vi "RFID GlobalVariable.vi"() -> ()   [LabVIEW 2018]
uses:
  Return_t.ctl
panel:
  out "_head":u16
  out "opcode Rd":u8 format="%x"
  out "crc Rd":u16=7439 format="%x"
  out "messageLength Rd":u8
  out "Wr Array":string[](array[string])
  out "msg read":u8[](array[numeric]) format="%x"
  in  "Tag Protocol":u16(ring)=5 items=["TMR_TAG_PROTOCOL_NONE"=0, "TMR_TAG_PROTOCOL_ISO180006B"=3, "TMR_TAG_PROTOCOL_GEN2"=5, "TMR_TAG_PROTOCOL_ISO180006B_UCODE"=6, "TMR_TAG_PROTOCOL_IPX64"=7, "TMR_TAG_PROTOCOL_IPX256"=8, "TMR_TAG_PROTOCOL_ATA"=29]
  in  "Region":u16(ring)=8 items=["REGION_INDIA"=4, "REGION_JAPAN"=5, "REGION_CHINA"=6, "REGION_EUROPE"=8, "REGION_KOREA"=9, "REGION_AUSTRALIA"=11, "REGION_NEWZEALAND"=13, "REGION_OPEN"=255]
  in  "Cmd_Time_Out":u16(ring)=2000 items=["COMMAND_TIME_OUT"=2000]
  in  "Opcode Constant":u16(ring) items=["TMR_SR_OPCODE_VERSION"=3, "TMR_SR_OPCODE_SET_BAUD_RATE"=6, "TMR_SR_OPCODE_READ_TAG_ID_SINGLE"=33, "TMR_SR_OPCODE_READ_TAG_ID_MULTIPLE"=34, "TMR_SR_OPCODE_WRITE_TAG_ID"=35, "TMR_SR_OPCODE_WRITE_TAG_DATA"=36, "TMR_SR_OPCODE_KILL_TAG"=38, "TMR_SR_OPCODE_READ_TAG_DATA"=40, "TMR_SR_OPCODE_CLEAR_TAG_ID_BUFFER"=42, "TMR_SR_OPCODE_MULTI_PROTOCOL_TAG_OP"=47, "TMR_SR_OPCODE_GET_READ_TX_POWER"=98, "TMR_SR_OPCODE_GET_WRITE_TX_POWER"=100, "TMR_SR_OPCODE_GET_POWER_MODE"=104, "TMR_SR_OPCODE_GET_READER_OPTIONAL_PARAMS"=106, "TMR_SR_OPCODE_GET_PROTOCOL_PARAM"=107, "TMR_SR_OPCODE_SET_ANTENNA_PORT"=145, "TMR_SR_OPCODE_SET_TAG_PROTOCOL"=147, "TMR_SR_OPCODE_SET_READ_TX_POWER"=146, "TMR_SR_OPCODE_SET_WRITE_TX_POWER"=148, "TMR_SR_OPCODE_SET_REGION"=151, "TMR_SR_OPCODE_SET_READER_OPTIONAL_PARAMS"=154, "TMR_SR_OPCODE_SET_PROTOCOL_PARAM"=155]
  in  "Return":T1
  out "opcode":u8 format="%x"
  out "crc":u16=7439 format="%x"
  out "messageLength":u8
  out "msg":u8[](array[numeric]) format="%x"
  # "Need only \nto debugging.\n<Arry of strings>"
  # "#define TMR_SR_OPCODE_VERSION 0x03\n#define TMR_SR_OPCODE_SET_BAUD_RATE 0x06\n#define TMR_SR_OPCODE_READ_TAG_ID_SINGLE 0x21\n#define TMR_SR_OPCODE_READ_TAG_ID_MULTIPLE 0x22\n#define TMR_SR_OPCODE_WRITE_TAG_ID 0x23\n#define TMR_SR_OPCODE_WRITE_TAG_DATA 0x24\n#define TMR_SR_OPCODE_KILL_TAG 0x26\n#define TMR_SR_OPCODE_READ_TAG_DATA 0x28\n#define TMR_SR_OPCODE_CLEAR_TAG_ID_BUFFER 0x2A\n#define TMR_SR_OPCODE_MULTI_PROTOCOL_TAG_OP 0x2F\n#define TMR_SR_OPCODE_GET_READ_TX_POWER 0x62\n#define TMR_SR_OPCODE_GET_WRITE_TX_POWER 0x64\n#define TMR_SR_OPCODE_GET_POWER_MODE 0x68\n#define TMR_SR_OPCODE_GET_READER_OPTIONAL_PARAMS 0x6A\n#define TMR_SR_OPCODE_GET_PROTOCOL_PARAM 0x6B\n#define TMR_SR_OPCODE_SET_ANTENNA_PORT 0x91\n#define TMR_SR_OPCODE_SET_TAG_PROTOCOL 0x93\n#define TMR_SR_OPCODE_SET_READ_TX_POWER 0x92\n#define TMR_SR_OPCODE_SET_WRITE_TX_POWER 0x94\n#define TMR_SR_OPCODE_SET_REGION 0x97\n#define TMR_SR_OPCODE_SET_READER_OPTIONAL_PARAMS 0x9A\n#define TMR_SR_OPCODE_SET_PROTOCOL_PARAM 0x9B"
  # "//Define all the ways functions can return\n#define ALL_GOOD 0\n#define ERROR_COMMAND_RESPONSE_TIMEOUT 1\n#define ERROR_CORRUPT_RESPONSE 2\n#define ERROR_WRONG_OPCODE_RESPONSE 3\n#define ERROR_UNKNOWN_OPCODE 4\n#define RESPONSE_IS_TEMPERATURE 5\n#define RESPONSE_IS_KEEPALIVE 6\n#define RESPONSE_IS_TEMPTHROTTLE 7\n#define RESPONSE_IS_TAGFOUND 8\n#define RESPONSE_IS_NOTAGFOUND 9\n#define RESPONSE_IS_UNKNOWN 10\n#define RESPONSE_SUCCESS 11\n#define RESPONSE_FAIL 12"
  # "#define REGION_INDIA 0x04\n#define REGION_JAPAN 0x05\n#define REGION_CHINA 0x06\n#define REGION_EUROPE 0x08\n#define REGION_KOREA 0x09\n#define REGION_AUSTRALIA 0x0B\n#define REGION_NEWZEALAND 0x0C\n#define REGION_NORTHAMERICA 0x0D\n#define REGION_OPEN 0xFF"
  # "//and possible future support\n//TMR_TAG_PROTOCOL_NONE              = 0x00\n//TMR_TAG_PROTOCOL_ISO180006B        = 0x03\n//TMR_TAG_PROTOCOL_GEN2              = 0x05\n//TMR_TAG_PROTOCOL_ISO180006B_UCODE  = 0x06\n//TMR_TAG_PROTOCOL_IPX64             = 0x07\n//TMR_TAG_PROTOCOL_IPX256            = 0x08\n//TMR_TAG_PROTOCOL_ATA               = 0x1D"
  # "#define COMMAND_TIME_OUT 2000"
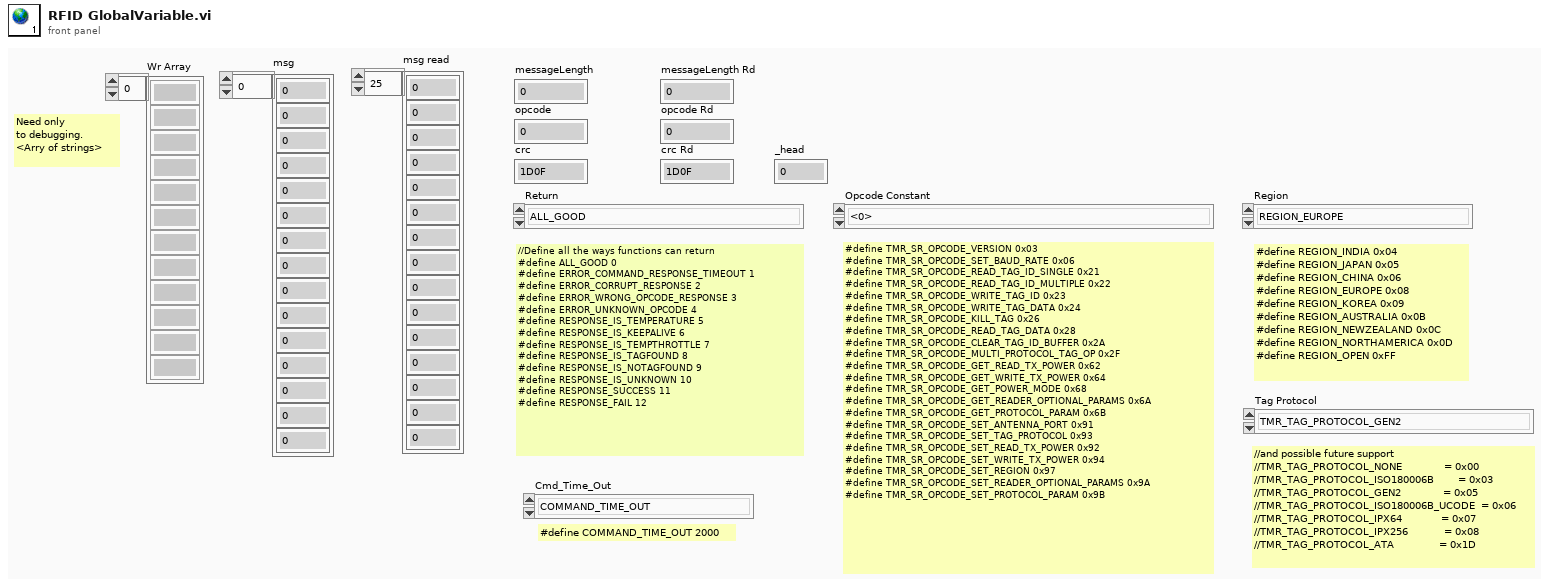
[diagram p1: front panel]
types:
  T1 = typedef "Return_t.ctl" = enum16{"ALL_GOOD", "ERROR_COMMAND_RESPONSE_TIMEOUT", "ERROR_CORRUPT_RESPONSE", "ERROR_WRONG_OPCODE_RESPONSE", "ERROR_UNKNOWN_OPCODE", "RESPONSE_IS_TEMPERATURE", "RESPONSE_IS_KEEPALIVE", "RESPONSE_IS_TEMPTHROTTLE", "RESPONSE_IS_TAGFOUND", "RESPONSE_IS_NOTAGFOUND", "RESPONSE_IS_UNKNOWN", "RESPONSE_SUCCESS", "RESPONSE_FAIL"}
diagram:
